vi "Arcade Mode.vi"(9 "Right Joystick":dbl(slide) scale=-1.0..1.0, 10 "Forward Joystick":dbl(slide) scale=-1.0..1.0) -> (1 "Right Power":dbl(slide) scale=-1.0..1.0, 2 "Left Power":dbl(slide) scale=-1.0..1.0)   [LabVIEW 2014, in "Driver.lvlib" / "Driver.lvclass"]
uses:
  Driver.lvclass
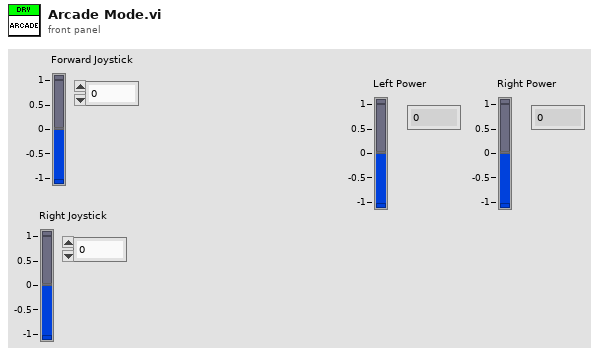
[diagram p1: front panel]
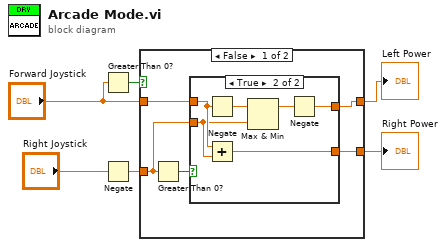
[diagram p0: block diagram]
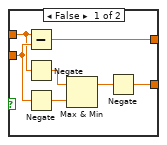
[diagram p2: hidden frame]
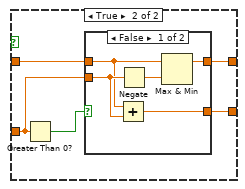
[diagram p3: hidden frame]
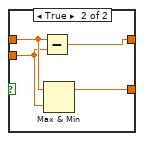
[diagram p4: hidden frame]
diagram:
  n1 = Greater Than 0?(x="Forward Joystick") -> (x > 0?=w6:bool)
  n2 = Negate(x="Right Joystick") -> (-x=w3:dbl)
  n3 = case shown="False" w6 {
    tunnel: w3 -> [w10 w28]
    tunnel: "Forward Joystick" -> [w9 w27]
    tunnel: [w8 w26] -> w5
    tunnel: [w7 w25] -> w4
    frame False {
      n4 = Greater Than 0?(x=w10) -> (x > 0?=w11:bool)
      n5 = case shown="True" w11 {
        tunnel: w10 -> [w18 w20]
        tunnel: w9 -> [w16 w21]
        tunnel: [w12 w22] -> w8
        tunnel: [w13 w19] -> w7
        frame False {
          n6 = Subtract(x=w16, y=w18) -> (x-y=w12:dbl)
          n7 = Negate(x=w16) -> (-x=w17:dbl)
          n8 = Negate(x=w18) -> (-x=w15:dbl)
          n9 = Max & Min(x=w17, y=w15) -> (max(x,y)=w14:dbl)  [unwired: 1 out]
          n10 = Negate(x=w14) -> (-x=w13:dbl)
        }
        frame True {
          n11 = Negate(x=w21) -> (-x=w24:dbl)
          n12 = Add(x=w21, y=w20) -> (x+y=w19:dbl)
          n13 = Max & Min(x=w24, y=w20) -> (max(x,y)=w23:dbl)  [unwired: 1 out]
          n14 = Negate(x=w23) -> (-x=w22:dbl)
        }
      }
    }
    frame True {
      n15 = Greater Than 0?(x=w28) -> (x > 0?=w29:bool)
      n16 = case shown="False" w29 {
        tunnel: w28 -> [w34 w36]
        tunnel: w27 -> [w31 w37]
        tunnel: [w32 w35] -> w26
        tunnel: [w30 w38] -> w25
        frame False {
          n17 = Add(x=w31, y=w34) -> (x+y=w30:dbl)
          n18 = Negate(x=w34) -> (-x=w33:dbl)
          n19 = Max & Min(x=w31, y=w33) -> (max(x,y)=w32:dbl)  [unwired: 1 out]
        }
        frame True {
          n20 = Subtract(x=w37, y=w36) -> (x-y=w35:dbl)
          n21 = Max & Min(x=w37, y=w36) -> (max(x,y)=w38:dbl)  [unwired: 1 out]
        }
      }
    }
  }
  "Left Power" <- w5
  "Right Power" <- w4
